vi "Reg0Write UnitTest.vi"() -> ()   [LabVIEW 2018]
uses:
  Command/RFFE Command.lvclass
  Downloads/MIPI RFFE API/Controls/RFFE Commands Type Def.ctl
  Downloads/MIPI RFFE API/Controls/Write Data Strict Type Def.ctl
  Reg0Write/RFFE Reg0Write Command.lvclass
  C:/Users/semoore/Projects/mipi-rffe-labview-oop/Command/RFFE Command.lvclass
panel:
  out "x = y?":bool
  out "logical AND":bool
  out "error in (no error) 2":errorcluster
  in  "error in (no error)":errorcluster
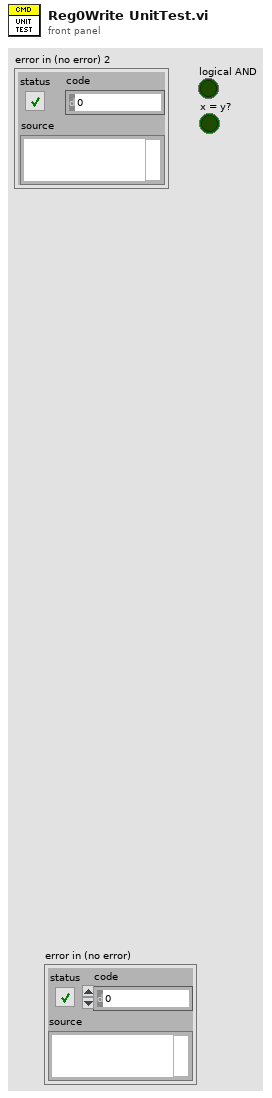
[diagram p1: front panel]
types:
  T1 = typedef "Write Data Strict Type Def.ctl" = cluster{"slave address":u8, "register address":u16, "register data (write)":u8[], "byte count":u8}
  T2 = typedef "RFFE Commands Type Def.ctl" = enum16{"Reg0Write", "RegWrite", "RegRead", "RegReadHR", "RegWriteExt", "RegReadExt", "RegReadExtHR", "RegWriteExtLong", "RegReadExtLong", "RegReadExtLongHR"}
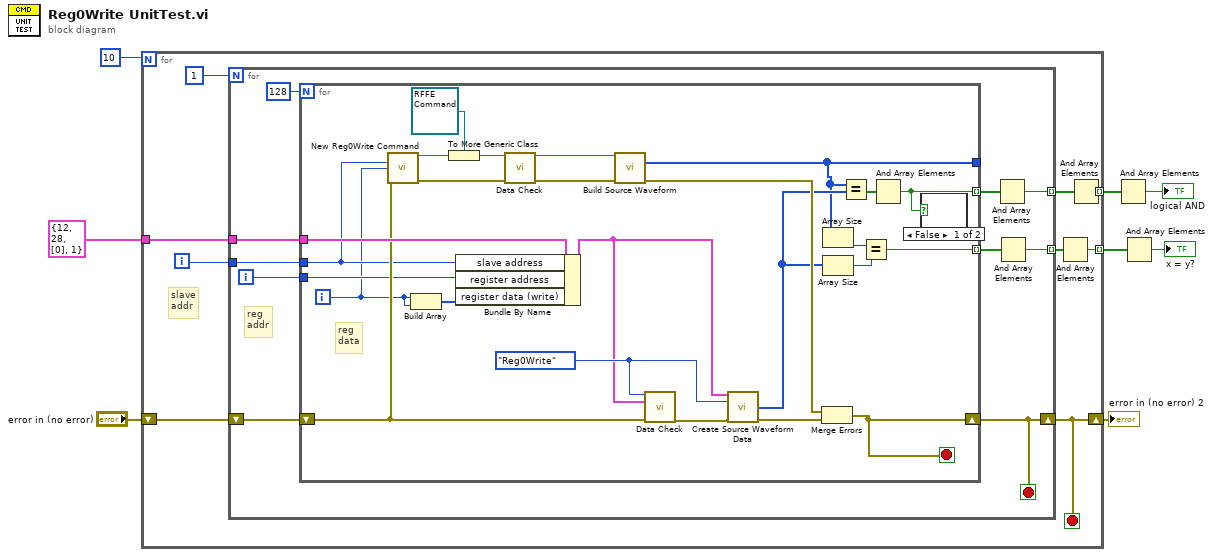
[diagram p0: block diagram]
diagram:
  n1 = for {
    N: 10 -> [_]
    tunnel: T1 {"slave address"=12, "register address"=28, "register data (write)"=[0], "byte count"=1} ("Register Data") -> [w16]
    shift-right: [w13] -> w5
    shift-left: "error in (no error)" -> [w17]
    tunnel: [w11] -> w4 mode=indexing
    tunnel: [w9] -> w2 mode=indexing
    i -> [w15]
    stop <- w13 stop-if-true
    # "slave\naddr"
    n2 = for {
      N: 1 -> [_]
      tunnel: w16 -> [w26]
      tunnel: w15 -> [w23]
      shift-right: [w22] -> w13
      shift-left: w17 -> [w27]
      tunnel: [w20] -> w12 mode=indexing
      tunnel: [w18] -> w10 mode=indexing
      i -> [w24]
      stop <- w22 stop-if-true
      # "reg\naddr"
      n3 = for {
        N: 128 -> [_]
        tunnel: w26 -> [w50]
        tunnel: [w33] -> _
        tunnel: w24 -> [w36]
        tunnel: w23 -> [w35]
        shift-right: [w40] -> w22
        shift-left: w27 -> [w37]
        tunnel: [w30] -> w21 mode=indexing
        tunnel: [w28] -> w19 mode=indexing
        i -> [w29]
        stop <- w40 stop-if-true
        w52 = RFFE_Commands_Type_Def."Reg0Write" ("RFFE command")
        # "reg\ndata"
        n4 = call "New Reg0Write Command.vi"("Slave Address"=w35, "Register Data"=w29, "error in (no error)"=w37) -> ("RFFE Reg0Write Command out"=w45:refnum<class "RFFE Reg0Write Command.lvclass">, "error out"=w47:errorcluster)  [unwired: 11 in]
        n5 = Build Array(w29, w29) -> (w42:i32[])
        n6 = To More Generic Class(target class=refnum<class "RFFE Command.lvclass"> refnum ("RFFE Commands.lvlib:RFFE Command.lvclass"), reference=w45) -> (generic class reference=w46:refnum<class "RFFE Command.lvclass">)
        n7 = Bundle By Name(cluster=w50, "slave address"=w35, "register address"=w36, "register data (write)"=w42) -> (w49:T1)
        n8 = call-dynamic "Data Check.vi"("RFFE Command in"=w46, "error in (no error)"=w47) -> ("RFFE Command out"=w44:refnum<class "RFFE Command.lvclass">, "error out"=w48:errorcluster)  [unwired: 12 in]
        n9 = call-dynamic "Build Source Waveform.vi"("RFFE Command in"=w44, "error in (no error)"=w48) -> ("Source Waveform"=w33:u32[], "error out"=w39:errorcluster)  [unwired: 11 in, 1 out]
        n10 = call "Data Check.vi"("RFFE command"=w52, "Register Data"=w49, "error in"=w37) -> ("error out"=w51:errorcluster)  [unwired: 12 in]
        n11 = call "Create Source Waveform Data.vi"("Register Data"=w49, "RFFE command"=w52, "error in"=w51) -> ("RFFEWrite source waveform data array"=w34:u32[], "error out"=w41:errorcluster)  [unwired: 10 in, 1 out]
        n12 = Merge Errors(w39, w41) -> (w40:errorcluster)
        n13 = Array Size(array=w33) -> (size(s)=w32:i32)
        n14 = Array Size(array=w34) -> (size(s)=w31:i32)
        n15 = Equal?(x=w33, y=w34) -> (x = y?=w38:bool[])
        n16 = Equal?(x=w32, y=w31) -> (x = y?=w28:bool)
        n17 = And Array Elements(Boolean array=w38) -> (logical AND=w30:bool)
        n18 = case shown="False" w30 {
          frame False {
          }
          frame True {
          }
        }
      }
      n19 = And Array Elements(Boolean array=w21) -> (logical AND=w20:bool)
      n20 = And Array Elements(Boolean array=w19) -> (logical AND=w18:bool)
    }
    n21 = And Array Elements(Boolean array=w10) -> (logical AND=w9:bool)
    n22 = And Array Elements(Boolean array=w12) -> (logical AND=w11:bool)
  }
  "error in (no error) 2" <- w5
  n23 = And Array Elements(Boolean array=w4) -> (logical AND=→"logical AND":bool)
  n24 = And Array Elements(Boolean array=w2) -> (logical AND=→"x = y?":bool)
